vi "ExampleWriter.vi"() -> ()   [LabVIEW 2011]
uses:
  0x2 Typedefs/RIO-OCU update controls.ctl
  2-Think/2 Typedefs/generalized sensor status.ctl
  2-Think/2 Typedefs/indicator LED.ctl
  2-Think/2 Typedefs/generalized actuator status.ctl
  2-Think/2 Typedefs/Which Boat.ctl
  2-Think/2 Typedefs/robot velocity.ctl
  2-Think/2 Typedefs/UTM Location.ctl
  2-Think/2 Typedefs/heading.ctl
  2-Think/2 Typedefs/rate of turn.ctl
  2-Think/2 Typedefs/pitch and roll.ctl
  2-Think/2 Typedefs/apparent wind.ctl
  2-Think/2 Typedefs/apparent wind speed.ctl
  2-Think/2 Typedefs/apparent wind direction.ctl
  2-Think/2 Typedefs/Velocity.ctl
  2-Think/2 Typedefs/absolute wind direction.ctl
  2-Think/2 Typedefs/absolute wind speed.ctl
  2-Think/2 Typedefs/absolute water current vector.ctl
  2-Think/2 Typedefs/rudder angle.ctl
  2-Think/2 Typedefs/sail setpt.ctl
  0x2 Typedefs/manual override.ctl
  2-Think/2 Typedefs/setpoints to boat.ctl
  0x2 Typedefs/Waypoints List.ctl
  0x2 Typedefs/ocuWaypoint.ctl
  0x2 Typedefs/waypointTypes.ctl
  0x2 Typedefs/Current Waypoint.ctl
  2-Think/2 Globals/2 Global.vi
  Writer/NetworkStreamWriter.lvclass
panel:
  in  "Monitored Items from RIO":T1 {"Robot Pitch/Roll"."Roll" format="%05.1f"; "Robot Pitch/Roll"."Pitch" format="%05.1f"; "Robot\nRate of Turn" format="%05.1f"; "Robot\nHeading" format="%05.1f"}
  out "Current iteration":i32
  in  "stop":bool
  # "How Am I?"
  # "Where Am I?"
  # "Path Planning"
  # "From Planning Functions"
  # "(this is not a cluster because subitems\nare generated in parallel code)"
  # "What's Around Me?"
  # "As Measured"
  # "As Measured"
  # "Loop Rates"
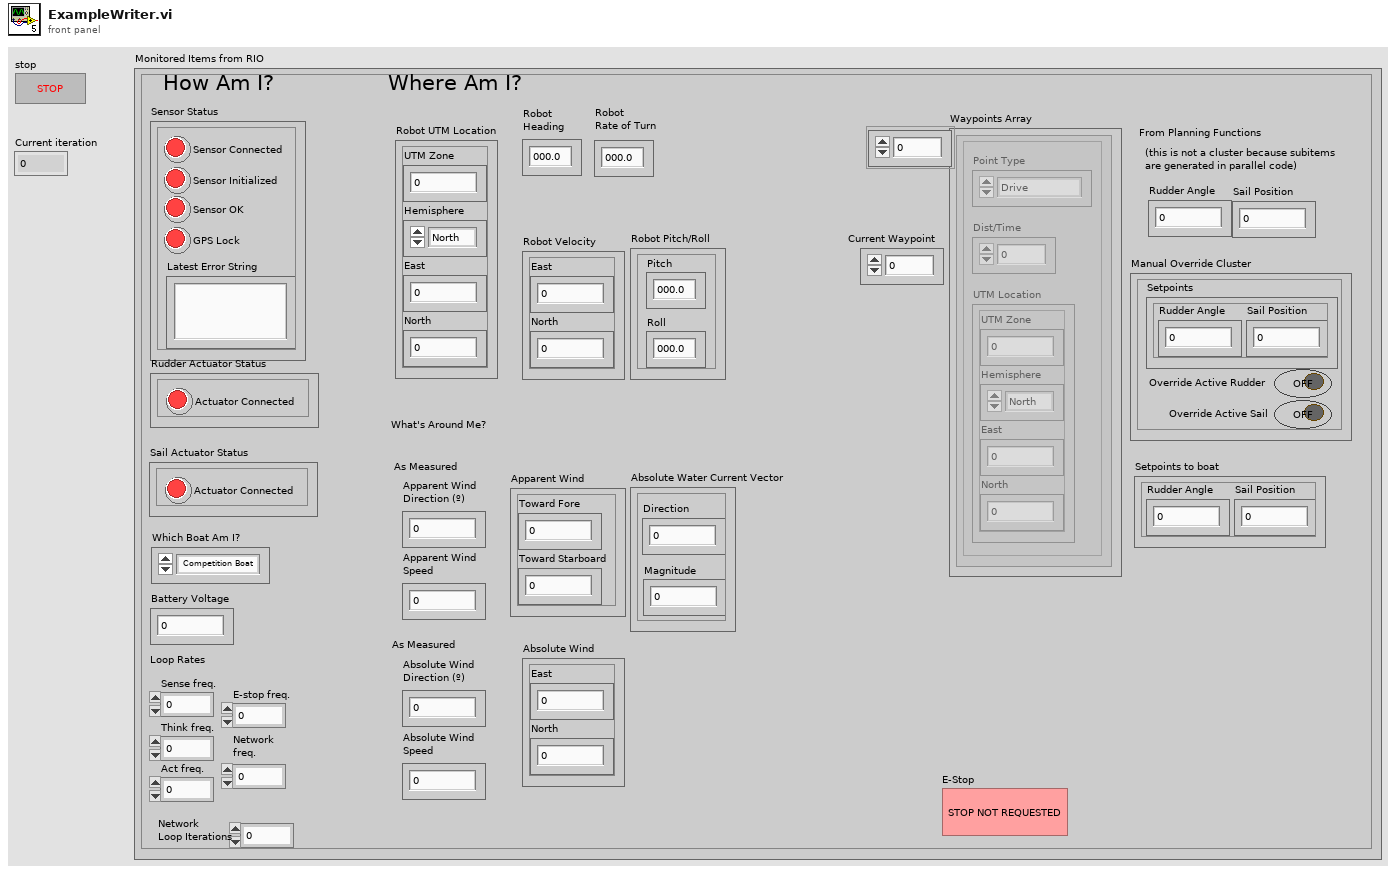
[diagram p1: front panel]
types:
  T1 = typedef "RIO-OCU update controls.ctl" = cluster{"Sensor Status":T2, "Battery Voltage":dbl, "Rudder Actuator Status":T4, "Sail Actuator Status":T4, "Which Boat Am I?":T5, "Robot Velocity":T6, "Robot UTM Location":T7, "Robot\nHeading ":T8, "Robot\nRate of Turn":T9, "Robot Pitch/Roll":T10, "Apparent Wind":T11, "Apparent Wind\nSpeed":T12, "Apparent Wind\nDirection (º)":T13, "Absolute Wind":T14, "Absolute Wind\nDirection (º)":T15, "Absolute Wind\nSpeed":T16, "Absolute Water Current Vector":T17, "Rudder Angle":T18, "Sail Position":T19, "Manual Override Cluster":T20, "Setpoints to boat":T21, "Waypoints Array":T22, "Current Waypoint":T25, "Think freq.":dbl, "Sense freq.":dbl, "Act freq.":dbl, "E-stop freq.":dbl, "Network \nfreq.":dbl, "Network \nLoop Iterations":i64, "E-Stop":bool}
  T2 = typedef "generalized sensor status.ctl" = cluster{"Sensor Connected":T3, "Sensor Initialized":T3, "Sensor OK":T3, "Latest Error String":string, "GPS Lock":T3}
  T3 = typedef "indicator LED.ctl" = bool
  T4 = typedef "generalized actuator status.ctl" = cluster{"Actuator Connected":T3}
  T5 = typedef "Which Boat.ctl" = enum16{"Competition Boat", "Small RC", "Simulation"}
  T6 = typedef "robot velocity.ctl" = cluster{"East":dbl, "North":dbl}
  T7 = typedef "UTM Location.ctl" = cluster{"UTM Zone":dbl, "Hemisphere":enum16{"North", "South"}, "East":dbl, "North":dbl}
  T8 = typedef "heading.ctl" = dbl
  T9 = typedef "rate of turn.ctl" = dbl
  T10 = typedef "pitch and roll.ctl" = cluster{"Pitch":dbl, "Roll":dbl}
  T11 = typedef "apparent wind.ctl" = cluster{"Toward Fore":dbl, "Toward Starboard":dbl}
  T12 = typedef "apparent wind speed.ctl" = dbl
  T13 = typedef "apparent wind direction.ctl" = dbl
  T14 = typedef "Velocity.ctl" = cluster{"East":dbl, "North":dbl}
  T15 = typedef "absolute wind direction.ctl" = dbl
  T16 = typedef "absolute wind speed.ctl" = dbl
  T17 = typedef "absolute water current vector.ctl" = cluster{"Direction":T13, "Magnitude":T13}
  T18 = typedef "rudder angle.ctl" = dbl
  T19 = typedef "sail setpt.ctl" = dbl
  T20 = typedef "manual override.ctl" = cluster{"Override Active Rudder":bool, "Setpoints":T21, "Override Active Sail":bool}
  T21 = typedef "setpoints to boat.ctl" = cluster{"Sail Position":T19, "Rudder Angle":T18}
  T22 = typedef "Waypoints List.ctl" = T23[]
  T23 = typedef "ocuWaypoint.ctl" = cluster{"Point Type":T24, "Dist/Time":dbl, "UTM Location":T7}
  T24 = typedef "waypointTypes.ctl" = enum16{"Drive", "Round Port", "Round Starboard", "Stay"}
  T25 = typedef "Current Waypoint.ctl" = i32
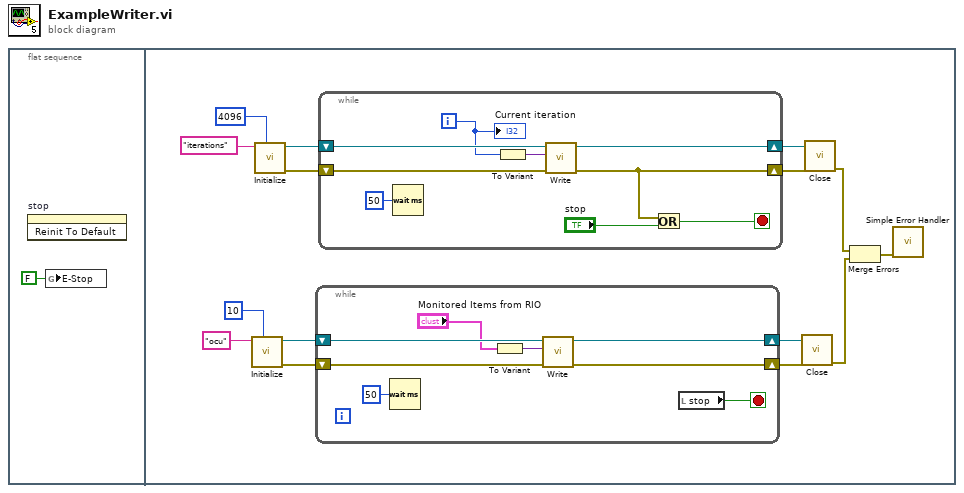
[diagram p0: block diagram]
diagram:
  n1 = flat-sequence {
    frame #0 {
      n2 = invoke on="stop" class="Bool (strict)" method="Reinit To Default"() -> ()  [unwired: 3 in, 3 out]
      n3 = global write "2 Global.vi" "E-Stop"(FALSE ("E-Stop")) -> ()
    }
    frame #1 {
      n4 = call "Initialize.vi"("writer buffer size"=10, "writer name"="ocu") -> ("error out"=w8:errorcluster, "NetworkStreamWriter out"=w7:refnum<class "NetworkStreamWriter.lvclass">)  [unwired: 8 in]
      n5 = call "Initialize.vi"("writer buffer size"=4096, "writer name"="iterations") -> ("error out"=w15:errorcluster, "NetworkStreamWriter out"=w16:refnum<class "NetworkStreamWriter.lvclass">)  [unwired: 8 in]
      n6 = while {
        shift-right: [w20] -> w11
        shift-left: w8 -> [w23]
        shift-right: [w22] -> w10
        shift-left: w7 -> [w24]
        stop <- w17 stop-if-true
        n7 = Wait (ms)(milliseconds to wait=u32 50) -> ()  [unwired: 1 out]
        n8 = To Variant(anything="Monitored Items from RIO") -> (Variant=w21:variant)
        n9 = call "Write.vi"("error in (no error)"=w23, "element"=w21, "NetworkStreamWriter in"=w24) -> ("error out"=w20:errorcluster, "NetworkStreamWriter out"=w22:refnum<class "NetworkStreamWriter.lvclass">)  [unwired: 7 in]
        n10 = local read "stop"() -> (w17:bool)
      }
      n11 = while {
        shift-right: [w28] -> w12
        shift-left: w15 -> [w32]
        shift-right: [w31] -> w13
        shift-left: w16 -> [w33]
        i -> [w30]
        stop <- w25 stop-if-true
        n12 = Wait (ms)(milliseconds to wait=u32 50) -> ()  [unwired: 1 out]
        n13 = To Variant(anything=w30) -> (Variant=w29:variant)
        n14 = call "Write.vi"("error in (no error)"=w32, "element"=w29, "NetworkStreamWriter in"=w33) -> ("error out"=w28:errorcluster, "NetworkStreamWriter out"=w31:refnum<class "NetworkStreamWriter.lvclass">)  [unwired: 7 in]
        n15 = Or(x=w28, y="stop") -> (x .or. y?=w25:bool)
        "Current iteration" <- w30
      }
      n16 = call "Close.vi"("error in (no error)"=w11, "NetworkStreamWriter in"=w10) -> ("error out"=w5:errorcluster)  [unwired: 8 in, 1 out]
      n17 = call "Close.vi"("error in (no error)"=w12, "NetworkStreamWriter in"=w13) -> ("error out"=w6:errorcluster)  [unwired: 8 in, 1 out]
      n18 = Merge Errors(w6, w5) -> (w4:errorcluster)
      n19 = call <vilib>:"Simple Error Handler.vi"("error in (no error)"=w4) -> ()  [unwired: 4 in, 5 out]
    }
  }
